vi "主程序.vi"() -> ()   [LabVIEW 2012]
panel:
  in  "数组":cluster{"x":dbl, "y":dbl}[](array[cluster])
  in  "图片":picture
  in  "状态":bool=TRUE
  in  "食物位置":cluster{"x":dbl, "y":dbl}
  in  "行列数":i32
  in  "点":cluster{"x":dbl, "y":dbl}
  in  "网格大小":dbl
  out "食物":bool
  in  "方向":i32
  out "new picture":picture
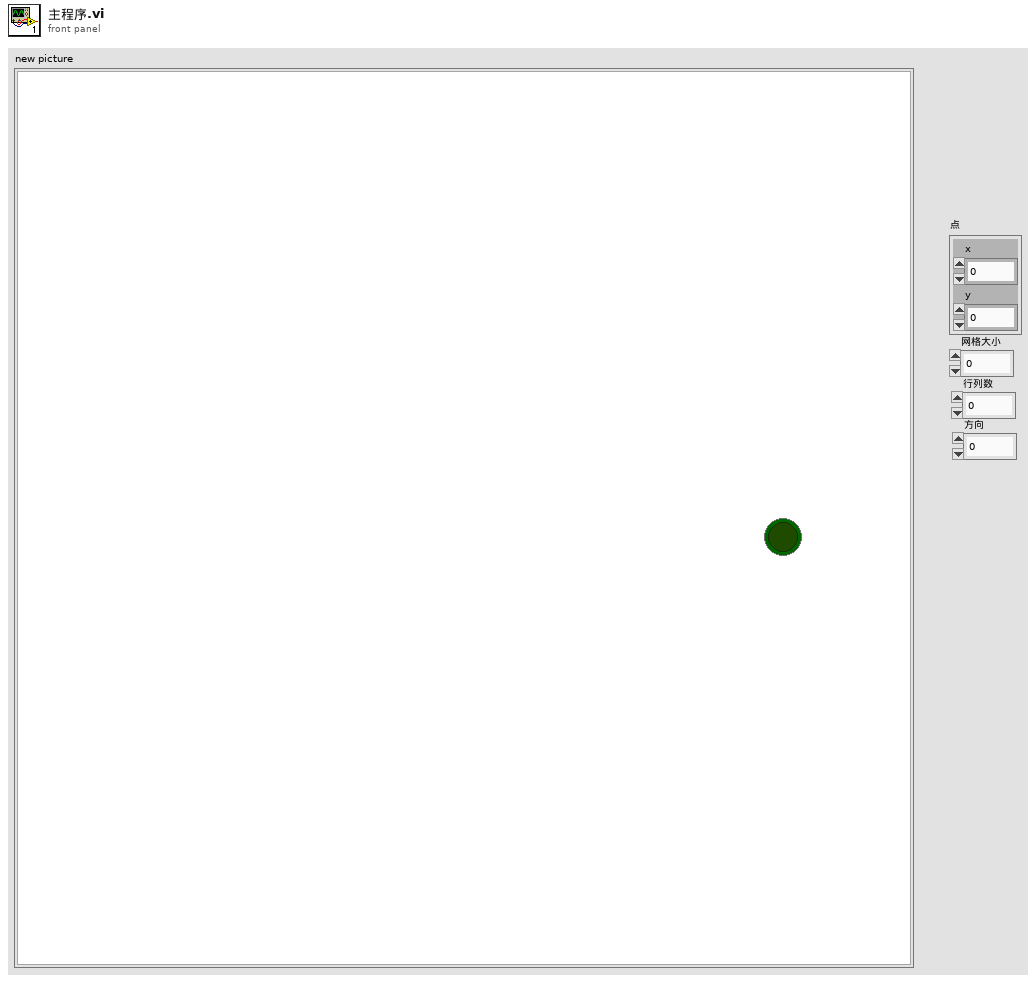
[diagram p1: front panel]
types:
  T1 = typedef "eventvkey.ctl" = enum16{"ASCII", "Enter", "Return", "Shift", "Ctrl", "Alt", "Cmd", "Opt", "Caps", "NumLock", "Clear", "Break", "Up", "Down", "Left", "Right", "Insert", "Delete", "Home", "End", "PageUp", "PageDown", "Escape", "Help", "Pause", "ScrollLock", "F1", "F2", "F3", "F4", "F5", "F6", "F7", "F8", "F9", "F10", "F11", "F12", "F13", "F14", "F15", "F16", "F17", "F18", "F19", "F20", "F21", "F22", "F23", "F24", "Play", "VolumeUp", "VolumeDown", "Mute", "Two Byte Char"}
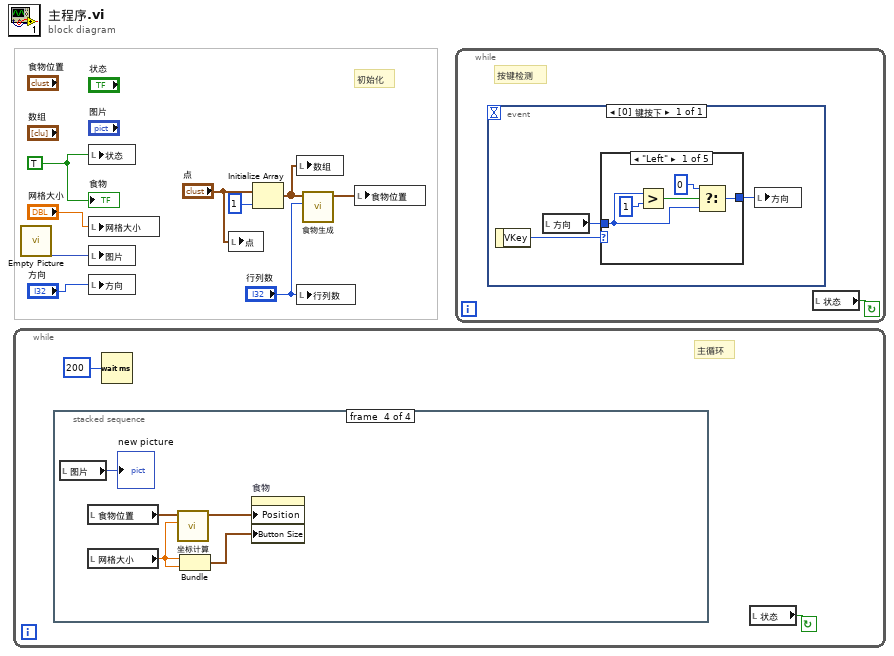
[diagram p0: block diagram]
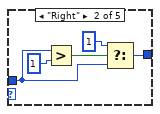
[diagram p2: hidden frame]
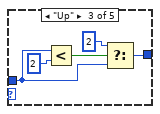
[diagram p3: hidden frame]
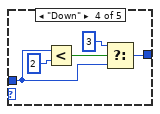
[diagram p4: hidden frame]
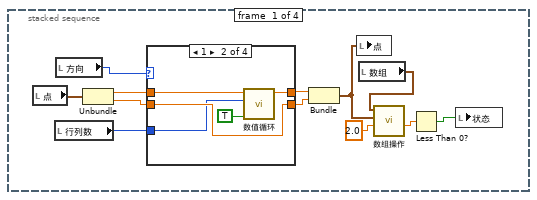
[diagram p6: hidden frame]
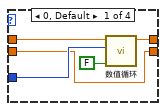
[diagram p7: hidden frame]
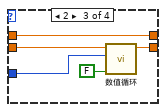
[diagram p8: hidden frame]
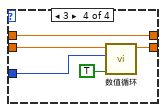
[diagram p9: hidden frame]
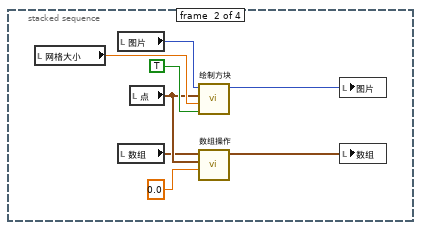
[diagram p10: hidden frame]
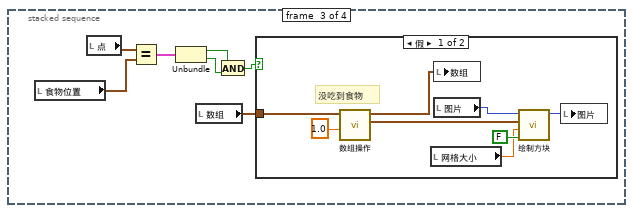
[diagram p11: hidden frame]
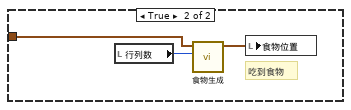
[diagram p12: hidden frame]
diagram:
  w2 = TRUE ("状态")
  # "初始化"
  n1 = while {
    stop <- w10 continue-if-true
    # "主循环"
    n2 = stacked-sequence {
      frame #0 {
        n3 = local read "点"() -> (w23:cluster{"x":dbl, "y":dbl})
        n4 = local read "行列数"() -> (w19:i32)
        n5 = local read "方向"() -> (w18:i32)
        n6 = Unbundle(w23) -> ("x"=w21:dbl, "y"=w20:dbl)
        n7 = case shown="1" w18 {
          tunnel: w21 -> [w28 w32 w36 w39]
          tunnel: w20 -> [w24 w30 w35 w42]
          tunnel: [w25 w31 w36 w39] -> w17
          tunnel: [w24 w30 w37 w40] -> w16
          tunnel: w19 -> [w26 w29 w34 w41]
          frame 0, Default {
            n8 = call "数值循环.vi"("加/减"=FALSE, "上限"=w26, "输入"=w28) -> ("输出"=w25:dbl)  [unwired: 8 in]
          }
          frame 1 {
            n9 = call "数值循环.vi"("加/减"=TRUE, "上限"=w29, "输入"=w32) -> ("输出"=w31:dbl)  [unwired: 8 in]
          }
          frame 2 {
            n10 = call "数值循环.vi"("加/减"=FALSE, "上限"=w34, "输入"=w35) -> ("输出"=w37:dbl)  [unwired: 8 in]
          }
          frame 3 {
            n11 = call "数值循环.vi"("加/减"=TRUE, "上限"=w41, "输入"=w42) -> ("输出"=w40:dbl)  [unwired: 8 in]
          }
        }
        n12 = Bundle("x"=w17, "输出"=w16) -> (w22:cluster{"x":dbl, "输出":dbl})  [unwired: 1 in]
        n13 = local write "点"(w22) -> ()
        n14 = local read "数组"() -> (w15:cluster{"x":dbl, "y":dbl}[])
        n15 = call "数组操作.vi"("操作码"=2.0, "输入点"=w22, "数组输入"=w15) -> ("索引"=w13:dbl)  [unwired: 6 in, 2 out]
        n16 = Less Than 0?(x=w13) -> (x < 0?=w12:bool)
        n17 = local write "状态"(w12) -> ()
      }
      frame #1 {
        n18 = local read "网格大小"() -> (w49:dbl)
        n19 = local read "图片"() -> (w48:picture)
        n20 = local read "数组"() -> (w45:cluster{"x":dbl, "y":dbl}[])
        n21 = local read "点"() -> (w46:cluster{"x":dbl, "y":dbl})
        n22 = call "绘制方块.vi"("绘制/清除"=TRUE, "网格大小"=w49, "输入点"=w46, "picture"=w48) -> ("new picture"=w47:picture)  [unwired: 7 in]
        n23 = call "数组操作.vi"("操作码"=0.0, "输入点"=w46, "数组输入"=w45) -> ("数组输出"=w44:cluster{"x":dbl, "y":dbl}[])  [unwired: 6 in, 2 out]
        n24 = local write "图片"(w47) -> ()
        n25 = local write "数组"(w44) -> ()
      }
      frame #2 {
        n26 = local read "食物位置"() -> (w58:cluster{"x":dbl, "y":dbl})
        n27 = local read "点"() -> (w56:cluster{"x":dbl, "y":dbl})
        n28 = Equal?(x=w56, y=w58) -> (x = y?=w57:cluster{"x":bool, "y":bool})
        n29 = Unbundle(w57) -> ("x"=w53:bool, "y"=w54:bool)
        n30 = local read "数组"() -> (w55:cluster{"x":dbl, "y":dbl}[])
        n31 = And(x=w53, y=w54) -> (x .and. y?=w52:bool)
        n32 = case shown="假" w52 {
          tunnel: w55 -> [w63 w67]
          frame False {
            # "没吃到食物"
            n33 = call "数组操作.vi"("操作码"=1.0, "数组输入"=w63) -> ("输出点"=w65:cluster{"x":dbl, "y":dbl}, "数组输出"=w60:cluster{"x":dbl, "y":dbl}[])  [unwired: 7 in, 1 out]
            n34 = local read "网格大小"() -> (w59:dbl)
            n35 = local write "数组"(w60) -> ()
            n36 = local read "图片"() -> (w62:picture)
            n37 = call "绘制方块.vi"("绘制/清除"=FALSE, "网格大小"=w59, "输入点"=w65, "picture"=w62) -> ("new picture"=w61:picture)  [unwired: 7 in]
            n38 = local write "图片"(w61) -> ()
          }
          frame True {
            # "吃到食物"
            n39 = local read "行列数"() -> (w68:i32)
            n40 = call "食物生成.vi"("上限"=w68, "数组输入"=w67) -> ("输出点"=w69:cluster{"x":dbl, "y":dbl})  [unwired: 9 in]
            n41 = local write "食物位置"(w69) -> ()
          }
        }
      }
      frame #3 {
        n42 = local read "图片"() -> (→"new picture":picture)
        n43 = local read "食物位置"() -> (w72:cluster{"x":dbl, "y":dbl})
        n44 = local read "网格大小"() -> (w73:dbl)
        n45 = call "坐标计算.vi"("网格大小"=w73, "输入"=w72) -> ("输出"=w71:cluster{"x":dbl, "y":dbl})  [unwired: 9 in]
        n46 = Bundle("网格大小"=w73, "网格大小"=w73) -> (w74:cluster{"网格大小":dbl, "网格大小":dbl})  [unwired: 1 in]
        n47 = property on="食物" class="Bool (严格)"("Position"=w71, "Button Size"=w74) -> ()  [unwired: 2 in, 2 out]
      }
    }
    n48 = Wait (ms)(milliseconds to wait=u32 200 ("等待时间（毫秒）")) -> ()  [unwired: 1 out]
    n49 = local read "状态"() -> (w10:bool)
  }
  n50 = call "Empty Picture"() -> ("empty picture"=w3:picture)
  n51 = local write "状态"(w2) -> ()
  n52 = local write "网格大小"("网格大小") -> ()
  n53 = local write "图片"(w3) -> ()
  n54 = local write "方向"("方向") -> ()
  n55 = local write "点"("点") -> ()
  n56 = Initialize Array("点", 1 ("维数大小")) -> (w5:cluster{"x":dbl, "y":dbl}[])
  n57 = local write "数组"(w5) -> ()
  n58 = local write "行列数"("行列数") -> ()
  n59 = call "食物生成.vi"("上限"="行列数", "数组输入"=w5) -> ("输出点"=w7:cluster{"x":dbl, "y":dbl})  [unwired: 9 in]
  n60 = local write "食物位置"(w7) -> ()
  n61 = while {
    stop <- w75 continue-if-true
    # "按键检测"
    n62 = event shown="[0] 键按下" {
      selector: _ -> [_]
      dyn-events: _ -> [_]
      timeout: _ -> [_]
      event Key Down {
        n63 = event-data() -> ("VKey"=w78:T1)  [unwired: 1 in]
        n64 = local read "方向"() -> (w77:i32)
        n65 = case shown="\"Left\"" w78 {
          tunnel: w77 -> [w80 w85 w90 w95 w99]
          tunnel: [w79 w84 w89 w94 w99] -> w76
          frame "Left" {
            n66 = Greater?(x=w80, y=1) -> (0:w82:bool)
            n67 = Select(t=u16 0, s=w82, f=w80) -> (s? t:f=w79:i32)
          }
          frame "Right" {
            n68 = Greater?(x=w85, y=1) -> (0:w87:bool)
            n69 = Select(t=u16 1, s=w87, f=w85) -> (s? t:f=w84:i32)
          }
          frame "Up" {
            n70 = Less?(x=w90, y=2) -> (x < y?=w92:bool)
            n71 = Select(t=u16 2, s=w92, f=w90) -> (s? t:f=w89:i32)
          }
          frame "Down" {
            n72 = Less?(x=w95, y=2) -> (x < y?=w97:bool)
            n73 = Select(t=u16 3, s=w97, f=w95) -> (s? t:f=w94:i32)
          }
          frame "ASCII", Default {
          }
        }
        n74 = local write "方向"(w76) -> ()
      }
    }
    n75 = local read "状态"() -> (w75:bool)
  }
  "食物" <- w2
